vi "PicoScope5000aGetValuesOverlappedBulk.vi"(5 "Segment Range":T1 {"toSegmentIndex" format="%.4p"; "fromSegmentIndex" format="%.4p"}, 7 "Buffer and Transfer Settings":T2={"startIndex"=0, "Samples"=1000, "Down Sample Ratio"=1, "Down-Sample Mode"=1} {"Down-Sample Mode" items=["None"=2147483648, "Aggregate"=1, "Decimate"=2, "Average"=4]; "Down Sample Ratio" step=1; "Samples" format="%_6p"}, 8 "error in (no error)":errorcluster, 11 "handle in":i16) -> (0 "error out":errorcluster, 3 "handle out":i16, 4 "Pointer to Overflow":u64[](array[numeric]), 6 "noOfSamples":u64)   [LabVIEW 2010]
doc: "Calls ps5000aGetValuesOverlappedBulk"
uses:
  ps5000a.dll
  shared/Buffer and Transfer Settings.ctl
  shared/Segment Range.ctl
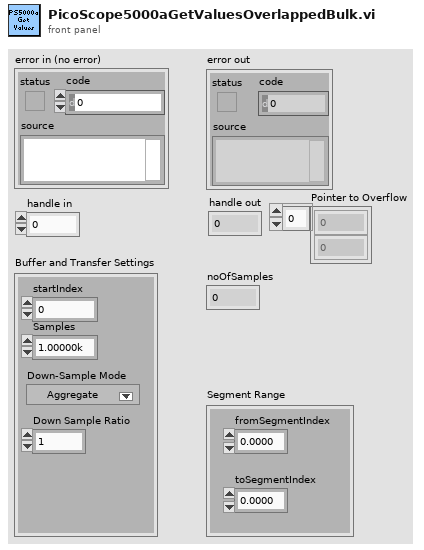
[diagram p1: front panel]
types:
  T1 = typedef "Segment Range.ctl" = cluster{"fromSegmentIndex":u64, "toSegmentIndex":u64}
  T2 = typedef "Buffer and Transfer Settings.ctl" = cluster{"startIndex":u64, "Samples":u64, "Down Sample Ratio":u64, "Down-Sample Mode":u32}
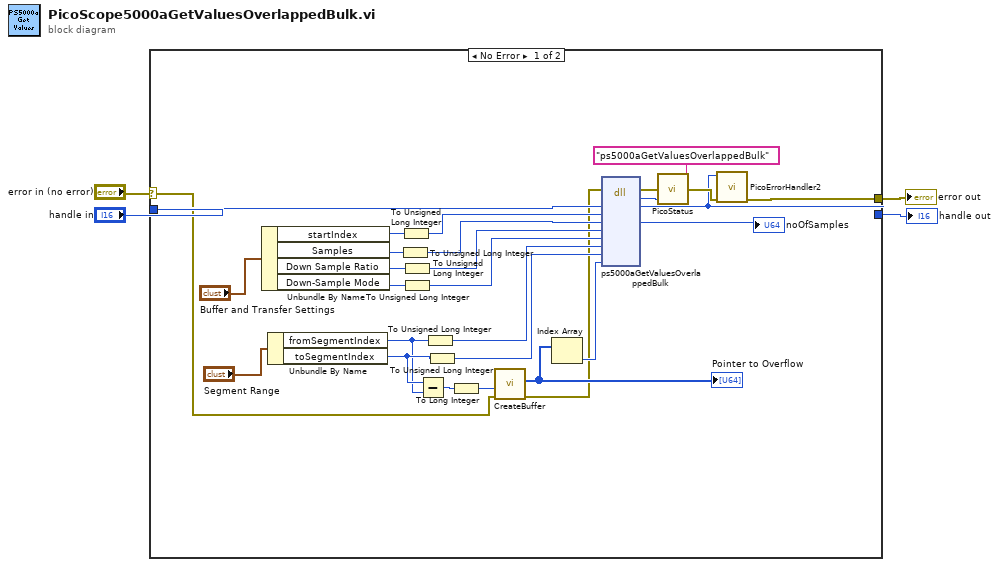
[diagram p0: block diagram]
diagram:
  n1 = case shown="No Error" "error in (no error)" {
    selector: "error in (no error)" -> [w5 w33]
    tunnel: "handle in" -> [w23 w34]
    tunnel: [w26 w34] -> w4
    tunnel: [w29 w33] -> w3
    frame No Error {
      n2 = Unbundle By Name("Buffer and Transfer Settings") -> ("startIndex"=w18:u64, "Samples"=w16:u64, "Down Sample Ratio"=w15:u64, "Down-Sample Mode"=w14:u32)
      n3 = Unbundle By Name("Segment Range") -> ("fromSegmentIndex"=w21:u64, "toSegmentIndex"=w22:u64)
      n4 = To Unsigned Long Integer(number=w16) -> (unsigned 32bit integer=w13:u32)
      n5 = To Unsigned Long Integer(number=w18) -> (unsigned 32bit integer=w17:u32)
      n6 = To Unsigned Long Integer(number=w15) -> (unsigned 32bit integer=w12:u32)
      n7 = To Unsigned Long Integer(number=w14) -> (unsigned 32bit integer=w11:u32)
      n8 = Subtract(x=w22, y=w21) -> (x-y=w24:u64)
      n9 = To Unsigned Long Integer(number=w21) -> (unsigned 32bit integer=w20:u32)
      n10 = To Unsigned Long Integer(number=w22) -> (unsigned 32bit integer=w19:u32)
      n11 = To Long Integer(number=w24) -> (32bit integer=w8:i32)
      n12 = call "CreateBuffer.vi"("error in (no error)"=w5, "Buffer size"=w8) -> ("error out"=w6:errorcluster, "Pointer and BufferSize"=w9:u64[])  [unwired: 8 in]
      "Pointer to Overflow" <- w9
      n13 = Index Array(array=w9) -> (element=w7:u64)  [unwired: 1 in]
      n14 = dll-call lib="ps5000a.dll" fn="ps5000aGetValuesOverlappedBulk" ("ps3000.dll:_ps3000_open_unit@0")(error in=w6, "handle"=w23, "startIndex"=w17, "noOfSamples"=w13, "downSampleRatio"=w12, "downSampleRatioMode"=w11, "fromSegmentIndex"=w20, "toSegmentIndex"=w19, "overflow"=w7) -> (error out=w27:errorcluster, "PICO_STATUS"=w25:u32, "handle"=w26:i16, "noOfSamples"=→"noOfSamples":u32)  [unwired: 8 in, 1 out]
      n15 = call "PicoStatus.vi"("PICO STATUS"=w25, "error in"=w27, "source"="ps5000aGetValuesOverlappedBulk") -> ("error out"=w32:errorcluster)
      n16 = call "PicoErrorHandler2.vi"("error in (no error)"=w32, "handle In"=w26) -> ("error out"=w29:errorcluster)  [unwired: 9 in]
    }
    frame Error {
    }
  }
  "error out" <- w3
  "handle out" <- w4
